vi "Water Tank Shell V1.vi"() -> ()   [LabVIEW 2018]
panel:
  out "Pos #2":bool
  out "Pos #1":bool
  in  "Heater":bool
  in  "Conveyor":bool
  in  "Pump":bool
  in  "Fill \nCup #2":bool
  in  "Fill \nCup #1":bool
  in  "Fill \nTank #2":bool
  in  "Fill \nTank #1":bool
  out "Auto/Manual":string
  in  "Auto/Manual":bool
  in  "Main Tank Set Level":dbl
  in  "Tank #2 Set Level":dbl
  out "Tank #2 Temp":dbl(slide) scale=0.0..150.0
  out "Main Tank Level":dbl(slide) scale=0.0..20.0
  in  "E Stop":bool
  out "Alerts":string
  out "Filling \nCup #2":bool
  out "Filling \nCup #1":bool
  out "Filling \nTank #2":bool
  out "Filling \nTank #1":bool
  in  "Temp Set Value":dbl
  in  "Tank #1 Set Level":dbl
  in  "Reset":bool
  in  "Start":bool
  out "Tank #1 Level":dbl(slide) scale=0.0..20.0
  out "Tank #2 Level":dbl(slide) scale=0.0..20.0
  out "Status":string
  in  "stop":bool
  out "Heater on":bool
  out "Conv on":bool
  out "Pump on":bool
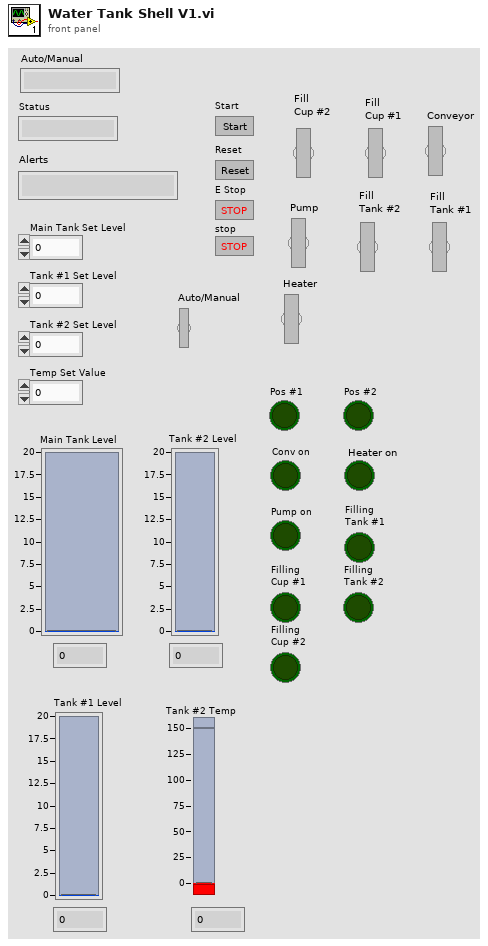
[diagram p1: front panel]
types:
  T1 = enum16{"Sate 0 Home", "State 1 Checking Main Tank", "State 2 Filling Tanks #1 & #2", "State 3 Moving to Position #1", "State 4 FillIng Cup #1 ", "State 5 Moving to Position #2", "State 6 Heating Tank #2", "State 7 Filling Cup #2", "State 8 Shutdown", "Manual"}
  T2 = cluster{"data[0]":bool, "data[1]":bool, "data[2]":bool, "data[3]":bool, "data[4]":bool, "data[5]":bool, "data[6]":bool, "data[7]":bool, "data[8]":bool}
  T3 = cluster{"Fill \nTank #1":bool, "Fill \nTank #2":bool, "Fill \nCup #1":bool, "Fill \nCup #2":bool, bool, "Pump":bool, "Conveyor":bool, "Heater":bool}
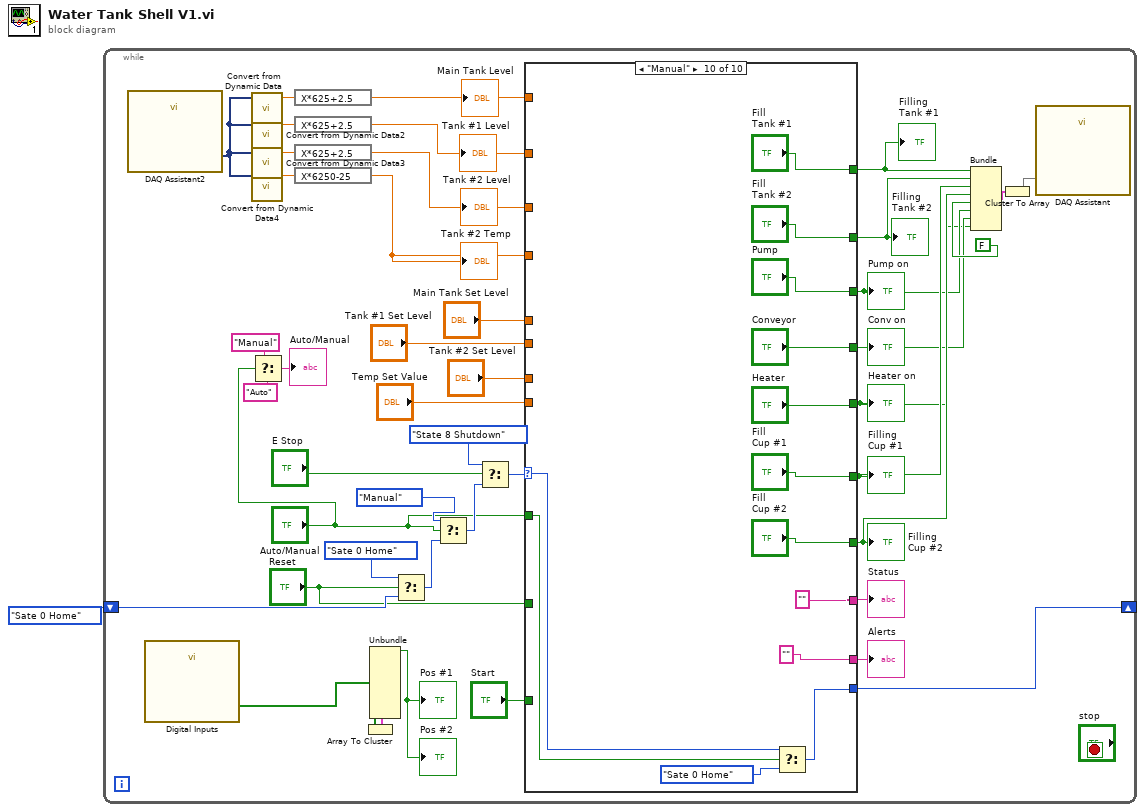
[diagram p0: block diagram]
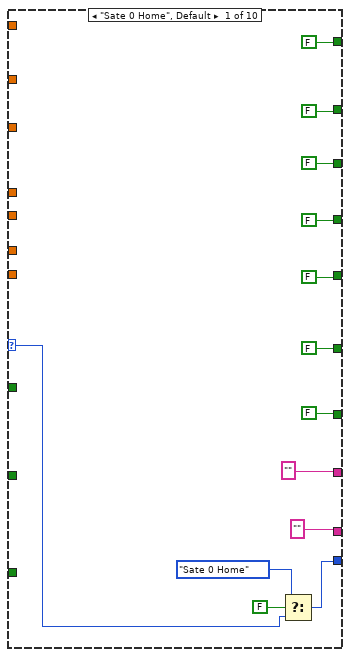
[diagram p2: hidden frame]
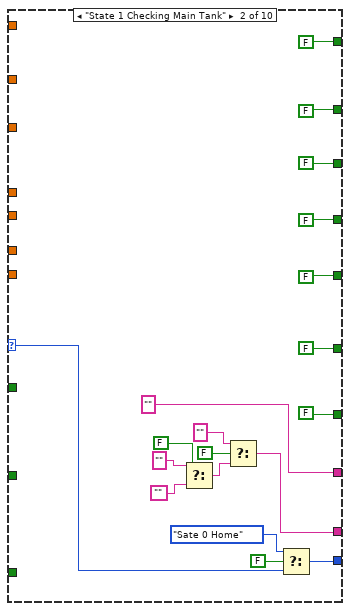
[diagram p3: hidden frame]
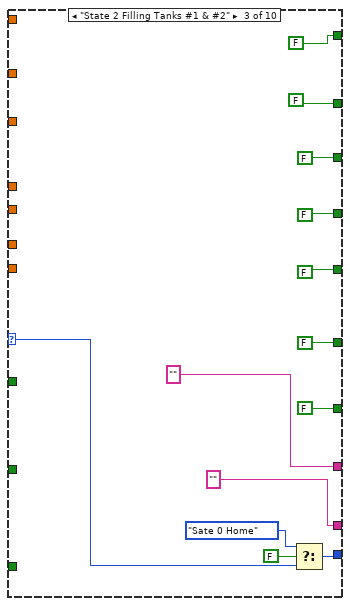
[diagram p4: hidden frame]
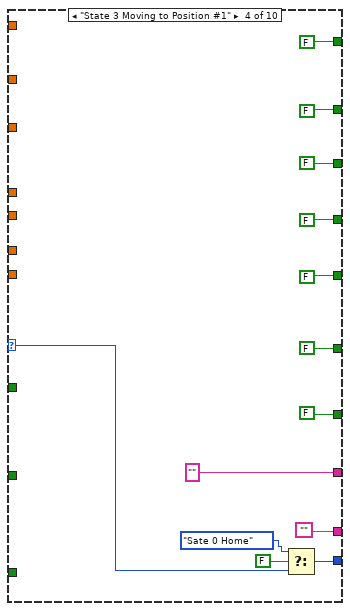
[diagram p5: hidden frame]
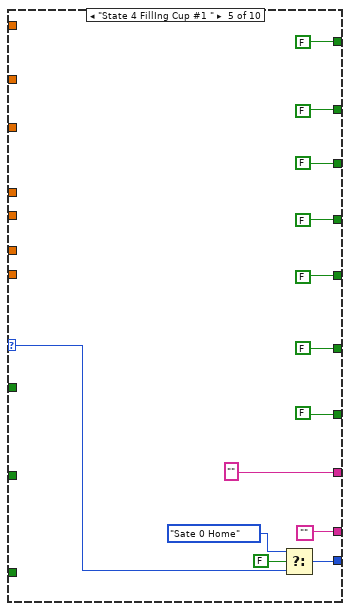
[diagram p6: hidden frame]
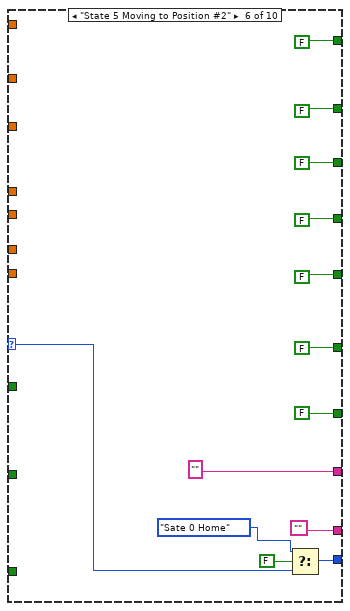
[diagram p7: hidden frame]
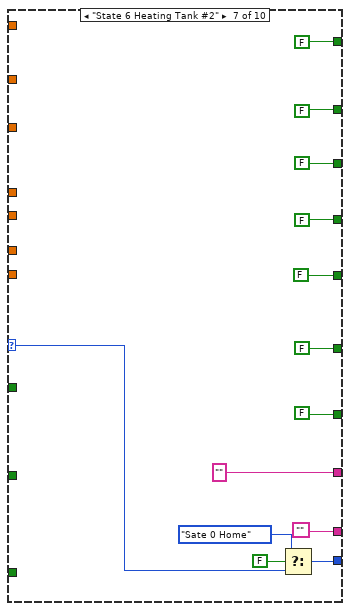
[diagram p8: hidden frame]
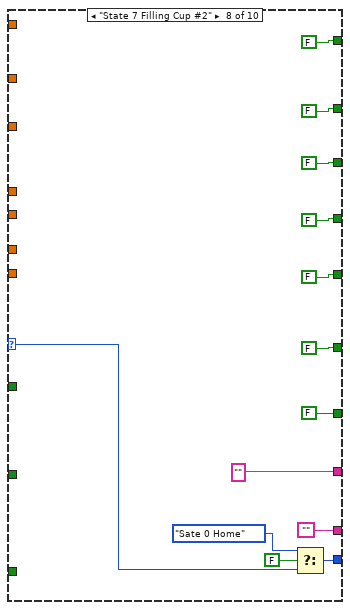
[diagram p9: hidden frame]
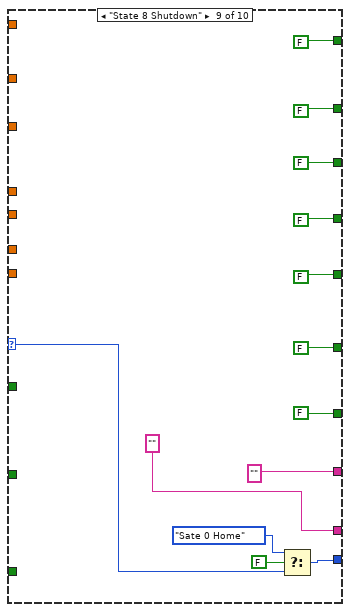
[diagram p10: hidden frame]
diagram:
  n1 = while {
    shift-right: [w41] -> _
    shift-left: T1."Sate 0 Home" -> [w20]
    stop <- "stop" stop-if-true
    n2 = call "DAQ Assistant2"() -> ("data"=w6:dynamicdata)  [unwired: 17 in, 2 out]
    n3 = call "Digital Inputs"() -> ("data"=w23:bool[])  [unwired: 17 in, 2 out]
    n4 = call "Convert from Dynamic Data"("Dynamic Data Type"=w6) -> ("Scalar"=w24:dbl)  [unwired: 3 in]
    n5 = call "Convert from Dynamic Data2"("Dynamic Data Type"=w6) -> ("Scalar"=w35:dbl)  [unwired: 3 in]
    n6 = call "Convert from Dynamic Data3"("Dynamic Data Type"=w6) -> ("Scalar"=w34:dbl)  [unwired: 3 in]
    n7 = call "Convert from Dynamic Data4"("Dynamic Data Type"=w6) -> ("Scalar"=w30:dbl)  [unwired: 3 in]
    n8 = Select(t="Manual", s="Auto/Manual", f="Auto") -> (s? t:f=→"Auto/Manual":string)
    n9 = expression code="X*625+2.5"(w24) -> (w33:dbl)
    "Main Tank Level" <- w33
    n10 = expression code="X*625+2.5"(w35) -> (w32:dbl)
    "Tank #1 Level" <- w32
    n11 = expression code="X*625+2.5"(w34) -> (w31:dbl)
    "Tank #2 Level" <- w31
    n12 = expression code="X*6250-25"(w30) -> (w29:dbl)
    "Tank #2 Temp" <- w29
    n13 = Array To Cluster(array=w23) -> (cluster=w42:T2)
    n14 = Unbundle(w42) -> ("data[0]"=→"Pos #1" →"Pos #2":bool)  [unwired: 8 out]
    n15 = Select(t=T1."Sate 0 Home", s="Reset", f=w20) -> (s? t:f=w21:T1)
    n16 = Select(t=T1."Manual", s="Auto/Manual", f=w21) -> (s? t:f=w22:T1)
    n17 = Select(t=T1."State 8 Shutdown", s="E Stop", f=w22) -> (s? t:f=w39:T1)
    n18 = case shown="\"Manual\"" w39 {
      selector: w39 -> [w49 w67 w83 w93 w106 w119 w133 w145 w158 w179]
      tunnel: ["" "" "" "" "" "" "" "" "" ""] -> w44
      tunnel: [FALSE FALSE FALSE FALSE FALSE FALSE FALSE FALSE FALSE "Fill \nCup #1"] -> w14
      tunnel: [FALSE FALSE FALSE FALSE FALSE FALSE FALSE FALSE FALSE "Heater"] -> w9
      tunnel: [FALSE FALSE FALSE FALSE FALSE FALSE FALSE FALSE FALSE "Conveyor"] -> w10
      tunnel: [FALSE FALSE FALSE FALSE FALSE FALSE FALSE FALSE FALSE "Pump"] -> w11
      tunnel: "Start" -> [_ _ _ _ _ _ _ _ _ _]
      tunnel: [FALSE FALSE FALSE FALSE FALSE FALSE FALSE FALSE FALSE "Fill \nTank #1"] -> w16
      tunnel: [FALSE FALSE FALSE FALSE FALSE FALSE FALSE FALSE FALSE "Fill \nTank #2"] -> w15
      tunnel: [FALSE FALSE FALSE FALSE FALSE FALSE FALSE FALSE FALSE "Fill \nCup #2"] -> w13
      tunnel: [w50 w68 w84 w94 w107 w120 w134 w146 w159 w180] -> w41
      tunnel: "Main Tank Set Level" -> [_ _ _ _ _ _ _ _ _ _]
      tunnel: "Tank #2 Set Level" -> [_ _ _ _ _ _ _ _ _ _]
      tunnel: "Tank #1 Set Level" -> [_ _ _ _ _ _ _ _ _ _]
      tunnel: ["" w70 "" "" "" "" "" "" "" ""] -> w40
      tunnel: "Temp Set Value" -> [_ _ _ _ _ _ _ _ _ _]
      tunnel: "Auto/Manual" -> [_ _ _ _ _ _ _ _ _ w169]
      tunnel: w33 -> [_ _ _ _ _ _ _ _ _ _]
      tunnel: w32 -> [_ _ _ _ _ _ _ _ _ _]
      tunnel: w31 -> [_ _ _ _ _ _ _ _ _ _]
      tunnel: w29 -> [_ _ _ _ _ _ _ _ _ _]
      tunnel: "Reset" -> [_ _ _ _ _ _ _ _ _ _]
      frame "Sate 0 Home", Default {
        n19 = Select(t=T1."Sate 0 Home", s=FALSE, f=w49) -> (s? t:f=w50:T1)
      }
      frame "State 1 Checking Main Tank" {
        n20 = Select(t="", s=FALSE, f="") -> (s? t:f=w64:string)
        n21 = Select(t="", s=FALSE, f=w64) -> (s? t:f=w70:string)
        n22 = Select(t=T1."Sate 0 Home", s=FALSE, f=w67) -> (s? t:f=w68:T1)
      }
      frame "State 2 Filling Tanks #1 & #2" {
        n23 = Select(t=T1."Sate 0 Home", s=FALSE, f=w83) -> (s? t:f=w84:T1)
      }
      frame "State 3 Moving to Position #1" {
        n24 = Select(t=T1."Sate 0 Home", s=FALSE, f=w93) -> (s? t:f=w94:T1)
      }
      frame "State 4 FillIng Cup #1 " {
        n25 = Select(t=T1."Sate 0 Home", s=FALSE, f=w106) -> (s? t:f=w107:T1)
      }
      frame "State 5 Moving to Position #2" {
        n26 = Select(t=T1."Sate 0 Home", s=FALSE, f=w119) -> (s? t:f=w120:T1)
      }
      frame "State 6 Heating Tank #2" {
        n27 = Select(t=T1."Sate 0 Home", s=FALSE, f=w133) -> (s? t:f=w134:T1)
      }
      frame "State 7 Filling Cup #2" {
        n28 = Select(t=T1."Sate 0 Home", s=FALSE, f=w145) -> (s? t:f=w146:T1)
      }
      frame "State 8 Shutdown" {
        n29 = Select(t=T1."Sate 0 Home", s=FALSE, f=w158) -> (s? t:f=w159:T1)
      }
      frame "Manual" {
        n30 = Select(t=w179, s=w169, f=T1."Sate 0 Home") -> (s? t:f=w180:T1)
      }
    }
    "Pump on" <- w11
    "Conv on" <- w10
    "Heater on" <- w9
    "Status" <- w44
    "Filling \nTank #1" <- w16
    "Filling \nCup #1" <- w14
    "Filling \nCup #2" <- w13
    "Filling \nTank #2" <- w15
    "Alerts" <- w40
    n31 = Bundle("Fill \nTank #1"=w16, "Fill \nTank #2"=w15, "Fill \nCup #1"=w14, "Fill \nCup #2"=w13, FALSE, "Pump"=w11, "Conveyor"=w10, "Heater"=w9) -> (w8:T3)  [unwired: 1 in]
    n32 = Cluster To Array(cluster=w8) -> (array=w7:bool[])
    n33 = call "DAQ Assistant"("data"=w7) -> ()  [unwired: 17 in, 2 out]
  }
